vi "Read Log_.vi"(8 "error in (no error)":errorcluster, 11 "Processing in":refnum<class "Processing.lvclass">) -> (0 "error out":errorcluster, 2 "Log?":bool, 3 "Processing out":refnum<class "Processing.lvclass">)   [LabVIEW 2015, in "Processing.lvclass"]
uses:
  Processing.lvclass
  Processing.lvclass/Processing.ctl
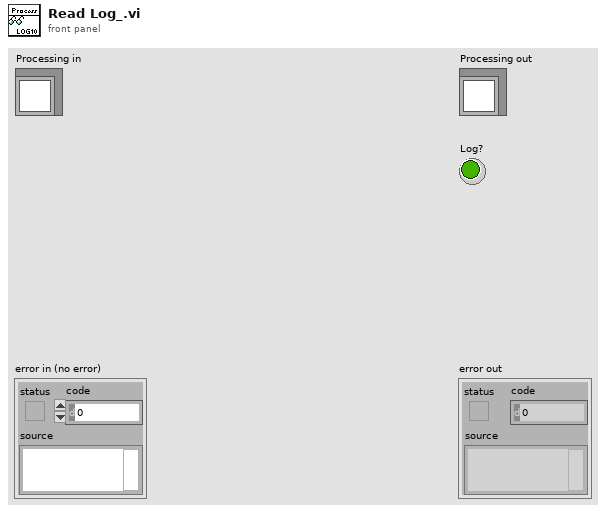
[diagram p1: front panel]
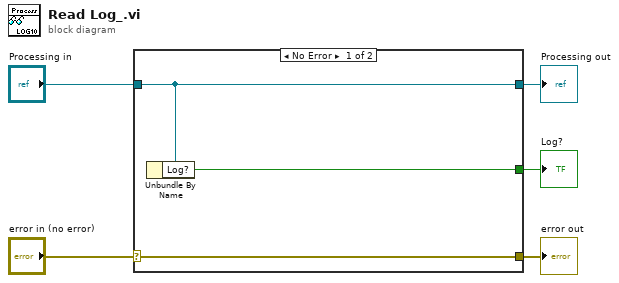
[diagram p0: block diagram]
diagram:
  n1 = case shown="No Error" "error in (no error)" {
    selector: "error in (no error)" -> [w8 w9]
    tunnel: [w8 w9] -> w4
    tunnel: [w7 w10] -> w2
    tunnel: "Processing in" -> [w7 w10]
    tunnel: [w6 _] -> w1
    frame No Error {
      n2 = Unbundle By Name(w7) -> ("Log?"=w6:bool)
    }
    frame Error {
    }
  }
  "error out" <- w4
  "Processing out" <- w2
  "Log?" <- w1
